vi "Signal-error.vi"(8 "error in (no error)":errorcluster, 11 "Data in":T1) -> (0 "error out":errorcluster, 3 "Data out":T1)   [LabVIEW 2013, in "PowderDeposition.lvlib" / "PD-Main.lvclass"]
uses:
  PD-Main.lvclass
  Object-reference.ctl
  PD-Main.lvclass/PD-Main.ctl
  Read Error log.vi
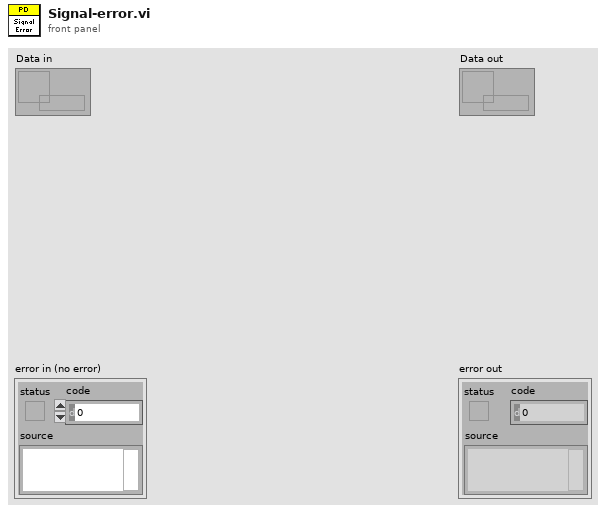
[diagram p1: front panel]
types:
  T1 = typedef "PowderDeposition.lvlib/PD-Main.lvclass/Object-reference.ctl" = refnum<data-value>
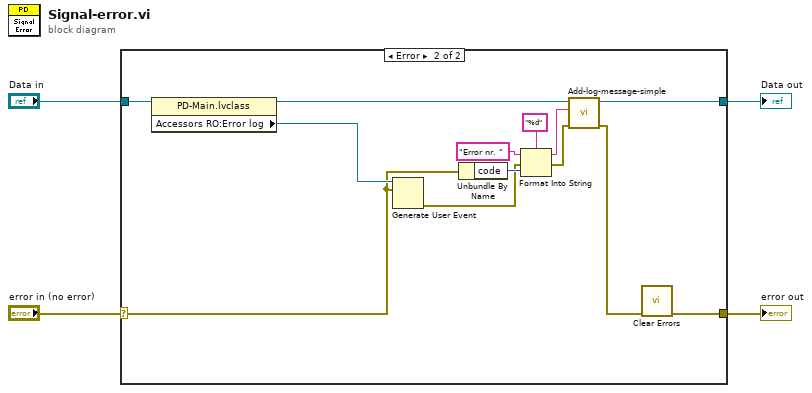
[diagram p0: block diagram]
diagram:
  n1 = case shown="Error" "error in (no error)" {
    selector: "error in (no error)" -> [w6 w9]
    tunnel: "Data in" -> [w5 w19]
    tunnel: [w5 w11] -> w3
    tunnel: [w6 w7] -> w2
    frame No Error {
    }
    frame Error {
      n2 = property class="PD-Main.lvclass"(reference=w19) -> (reference out=w12:T1, "Accessors RO:Error log"=w18:refnum<user-event>)  [unwired: 1 in, 1 out]
      n3 = Generate User Event(user event=w18, event data cluster=w9) -> (error out=w10:errorcluster)  [unwired: 2 in, 1 out]
      n4 = Unbundle By Name(w9) -> ("code"=w17:i32)
      n5 = Format Into String(format string="%d", initial string="Error nr. ", error in=w10, w17) -> (resulting string=w13:string, error out=w15:errorcluster)
      n6 = call "Add-log-message-simple.vi"("error in (no error)"=w15, "Message"=w13, "UI in"=w12) -> ("error out"=w8:errorcluster, "UI out"=w11:T1)  [unwired: 7 in]
      n7 = call <vilib>:"Clear Errors.vi"("error in (no error)"=w8) -> ("error out"=w7:errorcluster)  [unwired: 6 in]
    }
  }
  "error out" <- w2
  "Data out" <- w3
